vi "OneBallAuton.vi"() -> ()   [LabVIEW 2014]
uses:
  Events.vi
  AutonVars.vi
panel:
  out "WaitTime":dbl=3000.0
  out "TimeDriveFoward":dbl=2000.0
  out "Backward Speed":dbl=-0.68
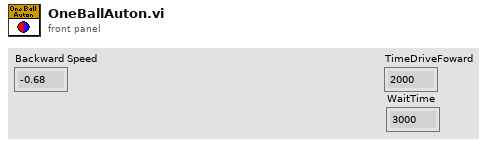
[diagram p1: front panel]
types:
  T1 = cluster{"Translate":dbl, "Y-Axis (Backward Speed)":dbl, "Rotate":dbl, "Tank right side":dbl, "axis 5":dbl, "axis 6":dbl, "Use gyro":bool, "Exponential\ndrive":bool, "Ring light":bool, "PID rotation":bool, "PID Gain":dbl}
  T2 = typedef "Eventgrab.ctl" = cluster{"Grab":bool, "GroundPass":bool, "Test Aqaure":dbl, "Shoulder up or down?":bool, "Auton drag":bool}
  T3 = cluster{"Reloading?":bool, "Throw":bool, "Ready?":bool, "Truss throw":bool, "Power is high?":bool, "Automatic relaod?":bool, "Manuall servo":bool}
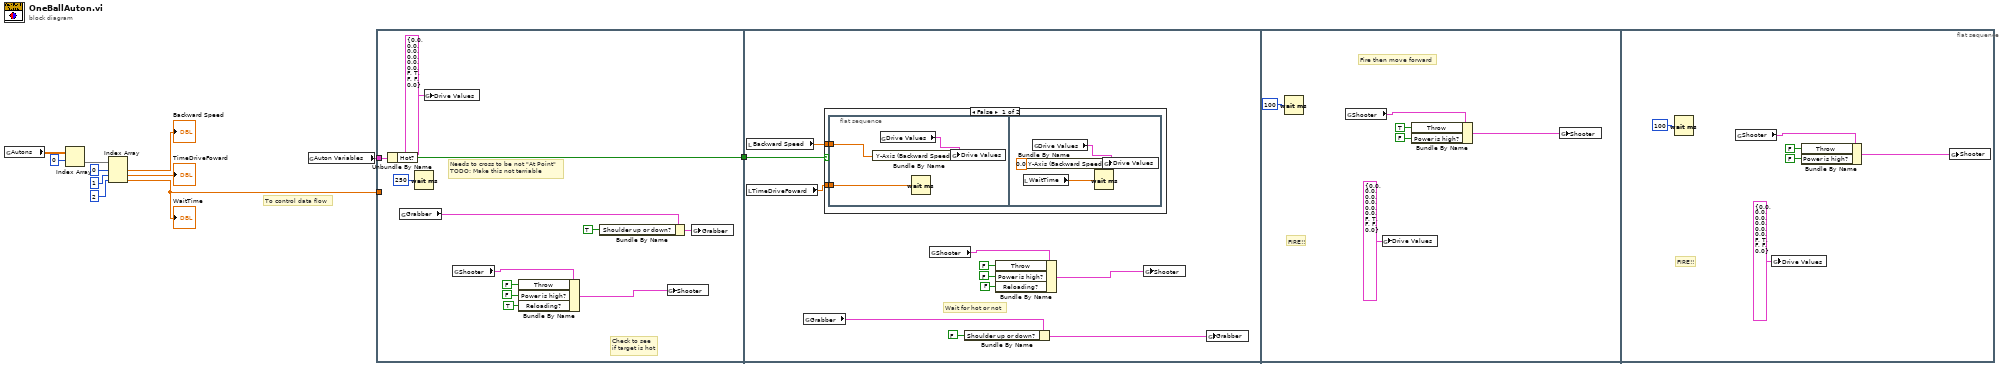
[diagram p0: block diagram]
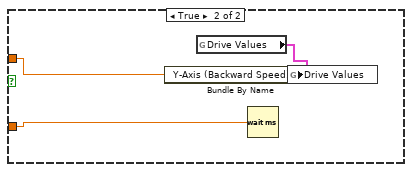
[diagram p2: hidden frame]
diagram:
  # "To control data flow"
  n1 = global read "AutonVars.vi" "Autons"() -> (w4:dbl[][])
  n2 = Index Array(array=w4, index (row)=0) -> (element=w2:dbl[])  [unwired: 1 in]
  n3 = Index Array(array=w2, index #1=0 ("index"), index #2=1 ("index"), index #3=2 ("index")) -> (element #1=→"Backward Speed":dbl, element #2=→"TimeDriveFoward":dbl, element #3=w1:dbl)
  "WaitTime" <- w1
  n4 = global read "Events.vi" "Auton Variables"() -> (w10:cluster{"Hot?":bool, "WhichAuton":string})
  n5 = flat-sequence {
    tunnel: [w23] -> w11
    tunnel: w10 -> [w21]
    tunnel: w1 -> [_]
    tunnel: w11 -> [w31]
    frame #0 {
      # "Needs to cross to be not \"At Point\"\nTODO: Make this not terriable"
      # "Check to see\nif target is hot"
      n6 = Unbundle By Name(w21) -> ("Hot?"=w23:bool)
      n7 = global read "Events.vi" "Grabber"() -> (w19:T2)
      n8 = Wait (ms)(milliseconds to wait=u32 250) -> ()  [unwired: 1 out]
      n9 = global write "Events.vi" "Drive Values"(T1 {"Translate"=0.0, "Y-Axis (Backward Speed)"=0.0, "Rotate"=0.0, "Tank right side"=0.0, "axis 5"=0.0, "axis 6"=0.0, "Use gyro"=FALSE, "Exponential\ndrive"=TRUE, "Ring light"=FALSE, "PID rotation"=FALSE, "PID Gain"=0.0} ("Drive Values")) -> ()
      n10 = global read "Events.vi" "Shooter"() -> (w17:T3)
      n11 = Bundle By Name(cluster=w17, "Throw"=FALSE, "Power is high?"=FALSE, "Reloading?"=TRUE) -> (w16:T3)
      n12 = Bundle By Name(cluster=w19, "Shoulder up or down?"=TRUE) -> (w18:T2)
      n13 = global write "Events.vi" "Shooter"(w16) -> ()
      n14 = global write "Events.vi" "Grabber"(w18) -> ()
    }
    frame #1 {
      # "Wait for hot or not"
      n15 = local read "TimeDriveFoward"() -> (w24:dbl)
      n16 = local read "Backward Speed"() -> (w25:dbl)
      n17 = global read "Events.vi" "Grabber"() -> (w33:T2)
      n18 = case shown="False" w31 {
        tunnel: w25 -> [w36 w46]
        tunnel: w24 -> [w35 w45]
        frame False {
          n19 = flat-sequence {
            tunnel: w36 -> [w38]
            tunnel: w35 -> [w37]
            frame #0 {
              n20 = global read "Events.vi" "Drive Values"() -> (w39:T1)
              n21 = Bundle By Name(cluster=w39, "Y-Axis (Backward Speed)"=w38) -> (w40:T1)
              n22 = Wait (ms)(milliseconds to wait=w37) -> ()  [unwired: 1 out]
              n23 = global write "Events.vi" "Drive Values"(w40) -> ()
            }
            frame #1 {
              n24 = local read "WaitTime"() -> (w41:dbl)
              n25 = global read "Events.vi" "Drive Values"() -> (w43:T1)
              n26 = Bundle By Name(cluster=w43, "Y-Axis (Backward Speed)"=0.0 ("Forward Speed")) -> (w44:T1)
              n27 = Wait (ms)(milliseconds to wait=w41) -> ()  [unwired: 1 out]
              n28 = global write "Events.vi" "Drive Values"(w44) -> ()
            }
          }
        }
        frame True {
          n29 = global read "Events.vi" "Drive Values"() -> (w47:T1)
          n30 = Bundle By Name(cluster=w47, "Y-Axis (Backward Speed)"=w46) -> (w48:T1)
          n31 = Wait (ms)(milliseconds to wait=w45) -> ()  [unwired: 1 out]
          n32 = global write "Events.vi" "Drive Values"(w48) -> ()
        }
      }
      n33 = global read "Events.vi" "Shooter"() -> (w30:T3)
      n34 = Bundle By Name(cluster=w33, "Shoulder up or down?"=FALSE) -> (w34:T2)
      n35 = Bundle By Name(cluster=w30, "Throw"=FALSE, "Power is high?"=FALSE, "Reloading?"=FALSE) -> (w29:T3)
      n36 = global write "Events.vi" "Shooter"(w29) -> ()
      n37 = global write "Events.vi" "Grabber"(w34) -> ()
    }
    frame #2 {
      # "FIRE!!"
      # "Fire then move forward"
      n38 = Wait (ms)(milliseconds to wait=u32 100) -> ()  [unwired: 1 out]
      n39 = global read "Events.vi" "Shooter"() -> (w54:T3)
      n40 = global write "Events.vi" "Drive Values"(T1 {"Translate"=0.0, "Y-Axis (Backward Speed)"=0.0, "Rotate"=0.0, "Tank right side"=0.0, "axis 5"=0.0, "axis 6"=0.0, "Use gyro"=FALSE, "Exponential\ndrive"=TRUE, "Ring light"=FALSE, "PID rotation"=FALSE, "PID Gain"=0.0} ("Drive Values")) -> ()
      n41 = Bundle By Name(cluster=w54, "Throw"=TRUE, "Power is high?"=FALSE) -> (w53:T3)
      n42 = global write "Events.vi" "Shooter"(w53) -> ()
    }
    frame #3 {
      # "FIRE!!"
      n43 = Wait (ms)(milliseconds to wait=u32 100) -> ()  [unwired: 1 out]
      n44 = global read "Events.vi" "Shooter"() -> (w60:T3)
      n45 = global write "Events.vi" "Drive Values"(T1 {"Translate"=0.0, "Y-Axis (Backward Speed)"=0.0, "Rotate"=0.0, "Tank right side"=0.0, "axis 5"=0.0, "axis 6"=0.0, "Use gyro"=FALSE, "Exponential\ndrive"=TRUE, "Ring light"=FALSE, "PID rotation"=FALSE, "PID Gain"=0.0} ("Drive Values")) -> ()
      n46 = Bundle By Name(cluster=w60, "Throw"=FALSE, "Power is high?"=FALSE) -> (w59:T3)
      n47 = global write "Events.vi" "Shooter"(w59) -> ()
    }
  }
